vi "MyG#G3Templ_Create.vi"(0 "reference in":refnum<class "MyG#G3Templ.lvclass">, 2 "MyAttribute":dbl, 5 "error in (no error)":errorcluster) -> (14 "reference out":refnum<class "MyG#G3Templ.lvclass">, 19 "error out":errorcluster)   [LabVIEW 2020, in "MyG#G3Templ.lvclass"]
doc: "Constructor."
uses:
  MyG#G3Templ.lvclass
  C:/Program Files (x86)/National Instruments/LabVIEW 2020/vi.lib/addons/_AddQ/G#Object/G#Object.lvclass
  vi.lib/addons/_AddQ/G#Object/G#Object.lvclass
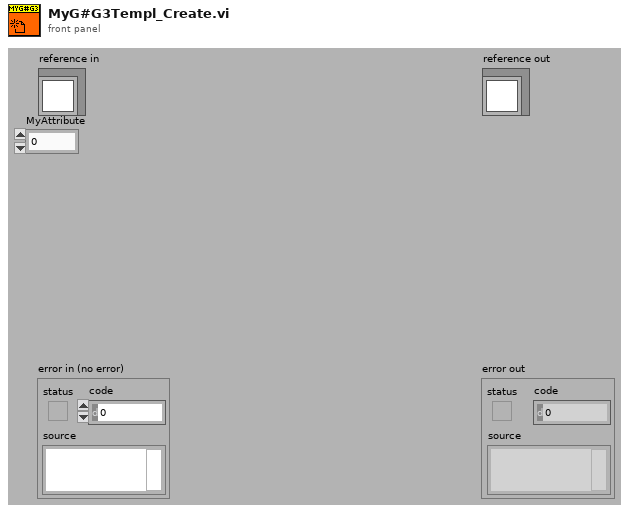
[diagram p1: front panel]
types:
  T1 = typedef "MyG#G3Templ.lvclass/ObjectAttributes.ctl" = cluster{"MyAttribute":dbl}
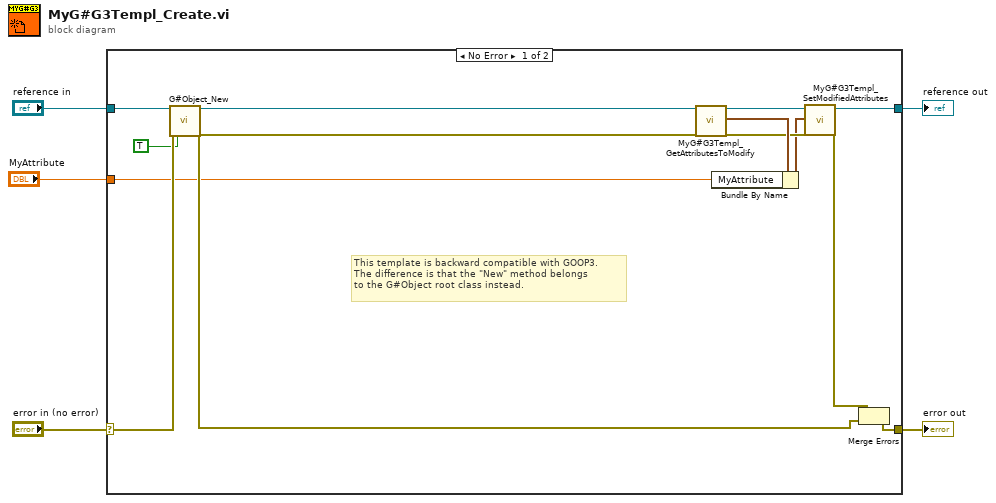
[diagram p0: block diagram]
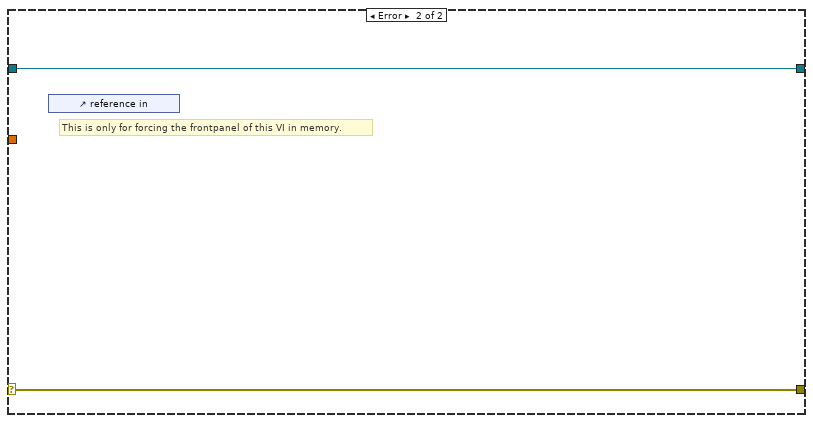
[diagram p2: hidden frame]
diagram:
  n1 = case shown="No Error" "error in (no error)" {
    selector: "error in (no error)" -> [w17 w20]
    tunnel: [w16 w20] -> w4
    tunnel: [w9 w19] -> w2
    tunnel: "reference in" -> [w18 w19]
    tunnel: "MyAttribute" -> [w6 _]
    frame No Error {
      # "This template is backward compatible with GOOP3.\nThe difference is that the \"New\" method belongs\nto the G#Object root class instead."
      n2 = call "G#Object_New.vi"("reference in"=w18, "error in (no error)"=w17, "user counter (T)?"=TRUE ("User Counter")) -> ("reference out"=w14:refnum<class "MyG#G3Templ.lvclass">, "error out"=w13:errorcluster)  [unwired: 14 in, 1 out]
      n3 = call "MyG#G3Templ_GetAttributesToModify.vi"("reference in"=w14, "error in (no error)"=w13) -> ("reference out"=w8:refnum<class "MyG#G3Templ.lvclass">, "attributes"=w12:T1, "error out"=w11:errorcluster)  [unwired: 13 in, 2 out]
      n4 = Bundle By Name(cluster=w12, "MyAttribute"=w6) -> (w7:T1)
      n5 = call "MyG#G3Templ_SetModifiedAttributes.vi"("reference in"=w8, "attributes"=w7, "error in (no error)"=w11) -> ("reference out"=w9:refnum<class "MyG#G3Templ.lvclass">, "error out"=w10:errorcluster)  [unwired: 15 in]
      n6 = Merge Errors(w10, w13) -> (w16:errorcluster)
    }
    frame Error {
      # "This is only for forcing the frontpanel of this VI in memory."
      n7 = control-ref of="reference in"() -> ()  [unwired: 1 out]
    }
  }
  "error out" <- w4
  "reference out" <- w2
